vi "数字波形的数据类型.vi"() -> ()   [LabVIEW 2010]
uses:
  <vilib>/Waveform/DWDTOps.llb/DWDT Analog to Digital.vi
  <vilib>/measure/NI_MABase.lvlib
panel:
  out "数字波形图":digitalwaveform[](graph)
  out "数字波形图":digitalwaveform(graph)
  out "数字波形图":cluster{i32, i32, i32[], i32}(graph)
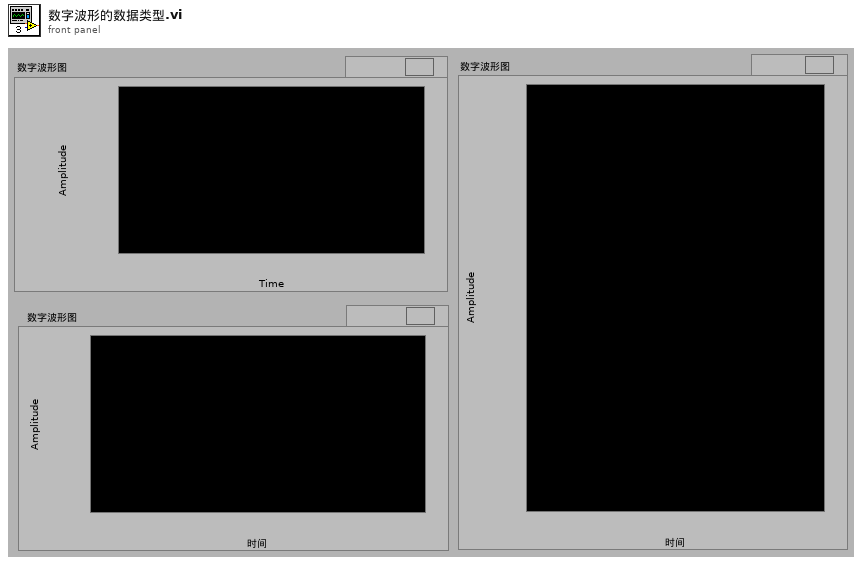
[diagram p1: front panel]
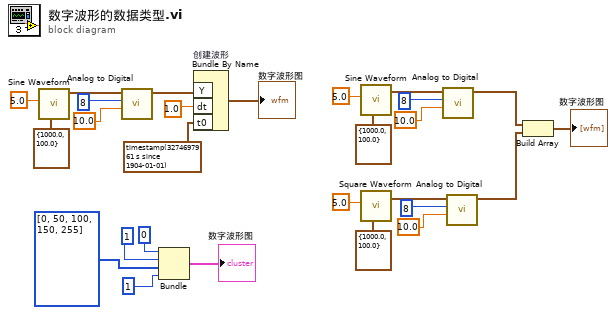
[diagram p0: block diagram]
diagram:
  n1 = call <vilib>:"Sine Waveform.vi"("sampling info"=cluster{"Fs":dbl, "#s":dbl} {"Fs"=1000.0, "#s"=100.0}, "amplitude"=5.0 ("Max (1.0)")) -> ("signal out"=w2:waveform(dbl))  [unwired: 8 in, 1 out]
  n2 = call-poly <vilib>:"Analog to Digital.vi"("full-scale range (pk-pk)"=10.0 ("Max (1.0)"), "resolution (16 bit)"=8 ("Resolution (16 bit)"), "analog waveform"=w2) -> ("digital waveform"=w1:digitalwaveform)  [unwired: 5 in, 3 out]
  n3 = Bundle(0, 1, i32[] [0, 50, 100, 150, 255], 1) -> (→"数字波形图":cluster{i32, i32, i32[], i32})  [unwired: 1 in]
  n4 = Bundle By Name "创建波形"("Y"=w1, "dt"=1.0, "t0"=timestamp(3274697961.59375 s since 1904-01-01)) -> (→"数字波形图":digitalwaveform)  [unwired: 1 in]
  n5 = call <vilib>:"Sine Waveform.vi"("sampling info"=cluster{"Fs":dbl, "#s":dbl} {"Fs"=1000.0, "#s"=100.0}, "amplitude"=5.0 ("Max (1.0)")) -> ("signal out"=w12:waveform(dbl))  [unwired: 8 in, 1 out]
  n6 = call <vilib>:"Square Waveform.vi"("sampling info"=cluster{"Fs":dbl, "#s":dbl} {"Fs"=1000.0, "#s"=100.0}, "amplitude"=5.0 ("Max (1.0)")) -> ("signal out"=w6:waveform(dbl))  [unwired: 8 in, 1 out]
  n7 = call-poly <vilib>:"Analog to Digital.vi"("full-scale range (pk-pk)"=10.0 ("Max (1.0)"), "resolution (16 bit)"=8 ("Resolution (16 bit)"), "analog waveform"=w12) -> ("digital waveform"=w11:digitalwaveform)  [unwired: 5 in, 3 out]
  n8 = call-poly <vilib>:"Analog to Digital.vi"("full-scale range (pk-pk)"=10.0 ("Max (1.0)"), "resolution (16 bit)"=8 ("Resolution (16 bit)"), "analog waveform"=w6) -> ("digital waveform"=w5:digitalwaveform)  [unwired: 5 in, 3 out]
  n9 = Build Array(w11, w5) -> (→"数字波形图":digitalwaveform[])
